vi "atidaqftmx.vi"() -> ()   [LabVIEW 2023]
doc: "I. Description:\nThis example demonstrates how to acquire a continuous amount of data (Waveform) using the DAQ device's internal clock.\n\nII. Instructions for Running:\n1. Create an analog input voltage channel.\n2. Set the rate for the sample clock. Additionally, define the sample mode to be continuous.\n3. Call the Start VI to start the acquisition.\n4. Read the waveform data in a loop until the user hits the stop button or an error occurs.\nNote: This example reads data from one or more channels and returns an array of data. Use the Index Array function to access an individual channel of data.\n5. Call the Clear Task VI to clear the Task.\n6. Use the popup dialog box to display an error if any.\n\nIV. I/O Connections Overview:\nMake sure your signal input terminal matches the Physical Channel I/O Control. For further connection information, refer to your hardware reference manual."
uses:
  <vilib>/Utility/error.llb/DialogType.ctl
  <vilib>/DAQmx/read.llb/DAQmx Read (Analog 2D DBL NChan NSamp).vi
  <vilib>/Analysis/baseanly.llb/A x Vector.vi
  <vilib>/DAQmx/create/channels.llb/DAQmx Create Channel (AI-Voltage-Basic).vi
  <vilib>/DAQmx/configure/timing.llb/DAQmx Timing (Sample Clock).vi
  <vilib>/DAQmx/miscellaneous.llb/DAQmx Fill In Error Info.vi
  <vilib>/Utility/file.llb/Write To Spreadsheet File (DBL).vi
  <vilib>/Analysis/NI_AALBase.lvlib
panel:
  in  "Torque Units":string
  in  "Force Units":string
  out "Torque Units":string
  out "Force Units":string
  in  "Transform":T1
  in  "Collect Data":bool=TRUE
  in  "Data File":path
  in  "Unbias":bool
  out "Bias Vector":dbl[](array[numeric])
  out "Bias Voltages":dbl[][](array[numeric])
  in  "Bias":bool
  out "Calibration Matrix":dbl[][](array[numeric])
  in  "Calibration File":path
  in  "stop":bool
  out "F/T":dbl[][](array[numeric]) format="%0.2f"
  out "Voltages":dbl[][](array[numeric])
  in  "First Channel":i16
  in  "DAQ Card":tag
  in  "Samples to Read":i32=1000
  in  "Minimum Value":dbl=-10.0 format="%0.2f"
  in  "Maximum Value":dbl=10.0 format="%0.2f"
  in  "Sample Rate":dbl=10000.0 caption="Sample Rate (Hz)" format="%0.2f"
  out "Measurement":dbl[][](graph) caption="F/T Data"
  # "Before running the VI, choose a data file to\nappend to.  While the VI is running, flip the\nswitch over to \"Collect Data\" to append\nforce and torque data to the file."
  # "Resolved Force/Torque Readings.  These are the first few \nrecords from the most recent set.  To see more records,\nexpand this array vertically, or set the major index."
  # "Make sure to choose a calibration\nfile before you start the VI.  The\nCalibration Index will almost\nalways be 1."
  # "Sensor Parameters"
  # "Fx"
  # "Fy"
  # "Fz"
  # "Tx"
  # "Ty"
  # "Tz"
  # "Enter Force and Torque units if\nyou want to output F/T values\nin different units than the\ncalibration. Leave blank to use\nthe units from the calibration."
  # "Stop Collecting Data"
  # "Channel Parameters"
  # "Select the NI-DAQmx board to\nwhich the sensor is connected,\nand the first channel the sensor\noccupies on that board.  If you\nare using a cable provided by\nATI, the first channel is most\nlikely 0.  If your sensor is\nconfigured for +/-5V, indicate\nthat here as well (most ATI\nsensors are configured for\n+/-10V)."
  # "Timing Parameters"
  # "Set the sample rate and the number of samples to read at\none time here.  The more samples you read at once, the\nlonger it will take to update the display.  However, reading\nlarge amounts of  data at once will free up more time to write\nthe data to the file and may prevent buffer overrun errors."
  # "These are the strain gauge values\nwhich are multiplied by the calibration\nmatrix to find the resolved force and\ntorque data."
  # "The calibration matrix is multiplied by the strain gauge voltage vector to find the\nresolved force and torque data.  Every sensor has a unique calibration matrix."
  # "This is the bias vector, which is the strain gauge reading that the\nsensor outputs when the sensor is unloaded, or when it is only\nloaded with something you wish to ignore the effects of."
  # "Input tool transform before starting VI to apply\na tool transformation to output F/T values.\n\nDisplacement values should be in the same units\nas the distance component of the torque units\nentered below the calibration file or the torque\nunits from the calibration if no units were specified\nabove. Rotation units are radians."
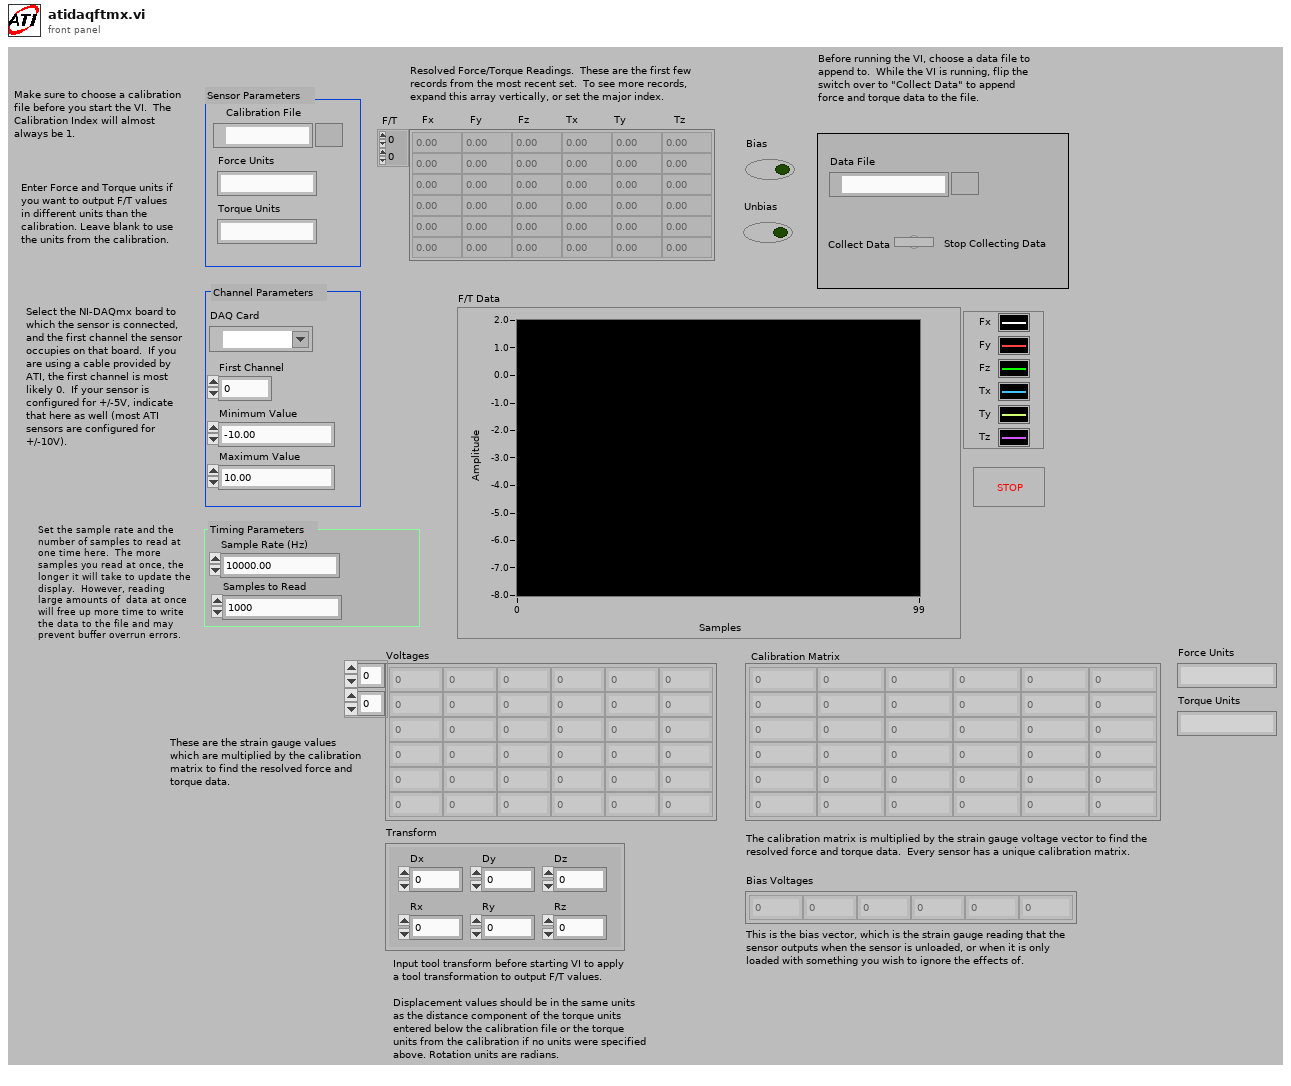
[diagram p1: front panel]
types:
  T1 = cluster{"Dx":dbl, "Dy":dbl, "Dz":dbl, "Rx":dbl, "Ry":dbl, "Rz":dbl}
  T2 = typedef "DialogType.ctl" = u16
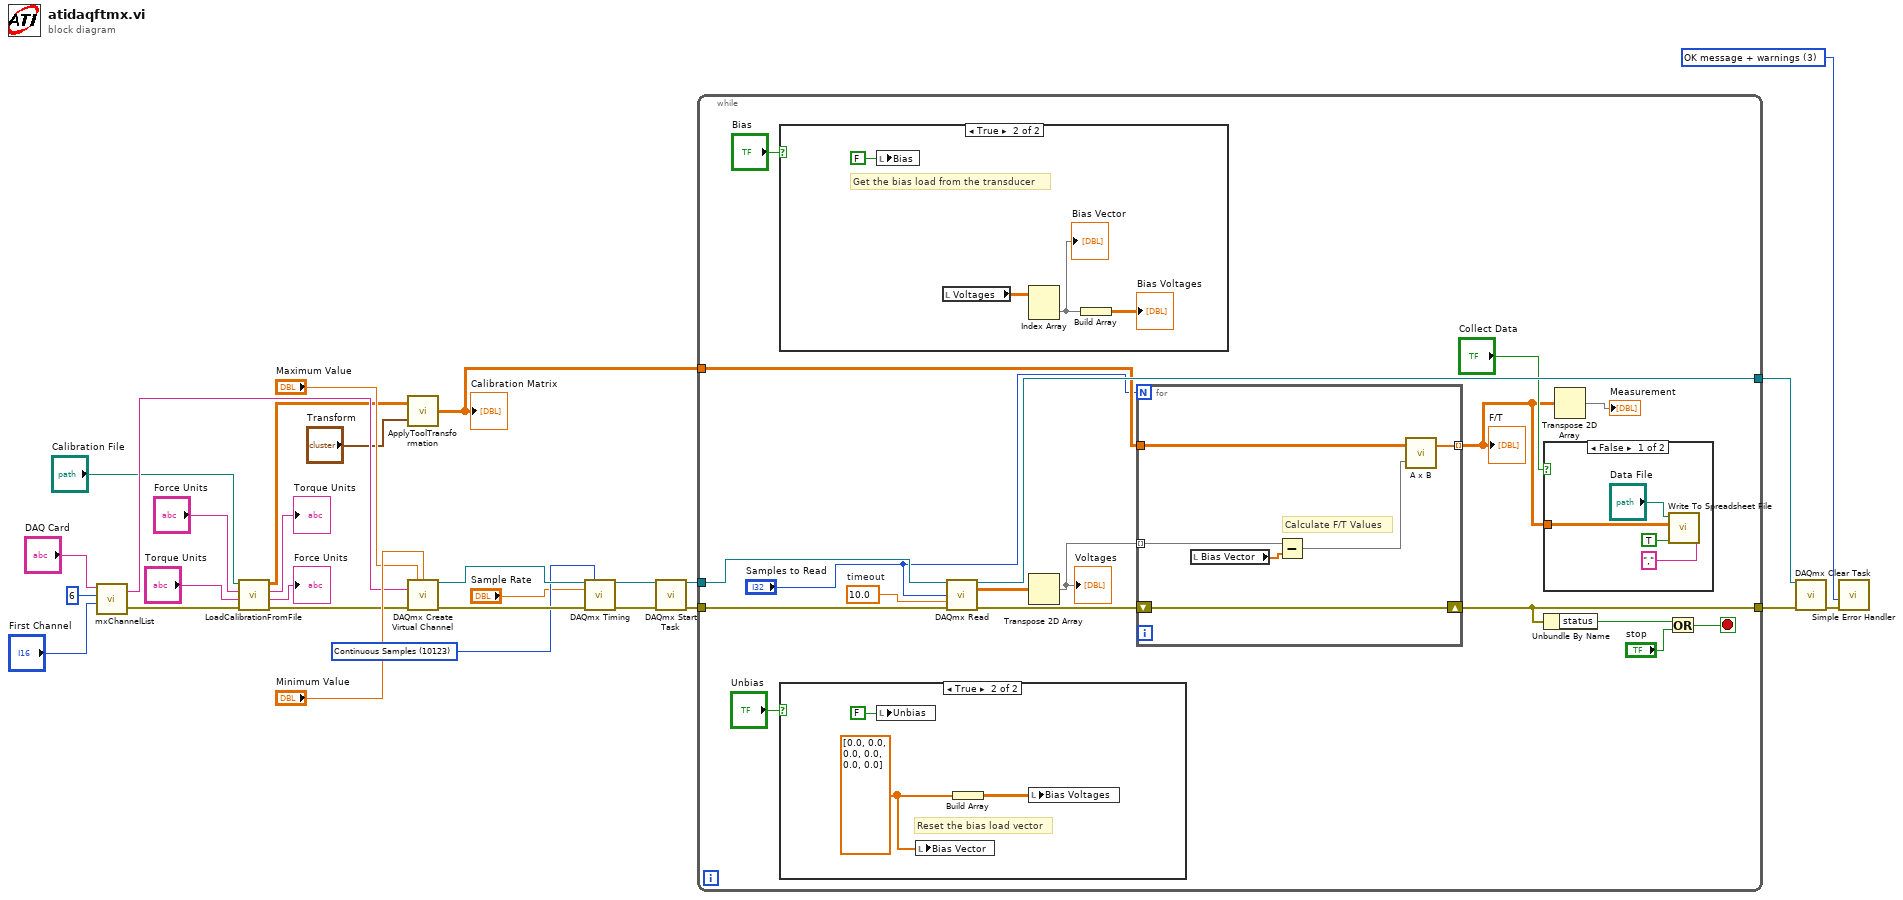
[diagram p0: block diagram]
diagram:
  w18 = T2 3 items=["no dialog", "OK message", "continue or stop message", "OK message + warnings", "continue/stop + warnings"] ("type of dialog (OK msg:1)")
  w21 = 10123 items=["Finite Samples"=10178, "Continuous Samples"=10123] ("sample mode")
  n1 = call "mxChannelList.vi"("First Channel"="First Channel", "Number of Channels"=6, "DAQmx Device Name"="DAQ Card") -> ("error out"=w2:errorcluster, "Channel List"=w14:string)  [unwired: 1 in]
  n2 = call "LoadCalibrationFromFile.vi"("Error In"=w2, "User Torque Units"="Torque Units", "User Force Units"="Force Units", "Cal File Path"="Calibration File") -> ("Error Out"=w1:errorcluster, "Calibration Force Units"=→"Force Units":string, "Calibration Torque Units"=→"Torque Units":string, "Calibration Matrix"=w8:dbl[][])
  n3 = call "ApplyToolTransformation.vi"("Transform"="Transform", "Calibration Matrix"=w8) -> ("Transformed Calibration Matrix"=w7:dbl[][])
  "Calibration Matrix" <- w7
  n4 = call-poly <vilib>:"DAQmx Create Virtual Channel.vi"("maximum value"="Maximum Value", "minimum value"="Minimum Value", "physical channels"=w14, "error in"=w1) -> ("task out"=w24:refnum<k21>, "error out"=w26:errorcluster)  [unwired: 10 in]
  n5 = call-poly <vilib>:"DAQmx Timing.vi"("task/channels in"=w24, "sample mode"=w21, "rate"="Sample Rate", "error in"=w26) -> ("task out"=w20:refnum<k21>, "error out"=w13:errorcluster)  [unwired: 10 in]
  n6 = call <vilib>:"DAQmx Start Task.vi"("task/channels in"=w20, "error in"=w13) -> ("task out"=w23:refnum<k21>, "error out"=w12:errorcluster)  [unwired: 12 in]
  n7 = while {
    tunnel: w23 -> [w46]
    tunnel: [w45] -> w22
    tunnel: w12 -> [w43]
    tunnel: [w38] -> w11
    tunnel: w7 -> [w35]
    stop <- w40 stop-if-true
    w44 = 10.0  # timeout
    n8 = case shown="True" "Bias" {
      frame False {
      }
      frame True {
        # "Get the bias load from the transducer"
        n9 = local write "Bias"(FALSE) -> ()
        n10 = local read "Voltages"() -> (w57:dbl[][])
        n11 = Index Array(array=w57) -> (element=w56:dbl[])  [unwired: 2 in]
        "Bias Vector" <- w56
        n12 = Build Array(w56) -> (→"Bias Voltages":dbl[][])
      }
    }
    n13 = case shown="True" "Unbias" {
      frame False {
      }
      frame True {
        w52 = dbl[] [0.0, 0.0, 0.0, 0.0, 0.0, 0.0]
        # "Reset the bias load vector"
        n14 = local write "Unbias"(FALSE) -> ()
        n15 = local write "Bias Vector"(w52) -> ()
        n16 = Build Array(w52) -> (w51:dbl[][])
        n17 = local write "Bias Voltages"(w51) -> ()
      }
    }
    n18 = call-poly <vilib>:"DAQmx Read.vi"("task/channels in"=w46, "number of samples per channel"="Samples to Read", "timeout"=w44, "error in"=w43) -> ("task out"=w45:refnum<k21>, "data"=w37:dbl[][], "error out"=w39:errorcluster)  [unwired: 9 in]
    n19 = Transpose 2D Array(2D array=w37) -> (transposed array=w33:dbl[][])
    "Voltages" <- w33
    n20 = for {
      N: "Samples to Read" -> [_]
      tunnel: [w60] -> w29 mode=indexing
      shift-right: [w59] -> w38
      shift-left: w39 -> [w59]
      tunnel: w33 -> [w63] mode=indexing
      tunnel: w35 -> [w58]
      # "Calculate F/T Values"
      n21 = local read "Bias Vector"() -> (w62:dbl[])
      n22 = Subtract(x=w63, y=w62) -> (x-y=w61:dbl[])
      n23 = call-poly <vilib>:"A x B.vi"("Vector"=w61, "A"=w58) -> ("A x Vector"=w60:dbl[])  [unwired: 1 out]
    }
    "F/T" <- w29
    n24 = case shown="False" "Collect Data" {
      tunnel: w29 -> [w50 _]
      frame False {
        n25 = call-poly <vilib>:"Write To Spreadsheet File.vi"("delimiter (\\t)"=",", "append to file? (new file:F)"=TRUE, "2D data"=w50, "file path (dialog if empty)"="Data File") -> ()  [unwired: 4 in, 1 out]
      }
      frame True {
      }
    }
    n26 = Unbundle By Name(w38) -> ("status"=w41:bool)
    n27 = Transpose 2D Array(2D array=w29) -> (transposed array=→"Measurement":dbl[][])
    n28 = Or(x=w41, y="stop") -> (x .or. y?=w40:bool)
  }
  n29 = call <vilib>:"DAQmx Clear Task.vi"("task in"=w22, "error in"=w11) -> ("error out"=w25:errorcluster)  [unwired: 13 in]
  n30 = call <vilib>:"Simple Error Handler.vi"("type of dialog (OK msg:1)"=w18, "error in (no error)"=w25) -> ()  [unwired: 3 in, 5 out]
